vi "Shrink blobs by N pixels.vi"(8 "error in (no error)":errorcluster, 9 "Pixels to shrink":dbl=10.0, 11 "Image In":T1) -> (0 "error out":errorcluster, 3 "Image out":T1)   [LabVIEW 2013]
doc: "This vi uses a Daniellson tranfomation of the drop binary image followed by a threshold to shrink the diameter of the drop mask. Any point originally part of the mask that is within \"pixels to shrink\" of the boarder is removed from the drop mask out."
uses:
  <vilib>/vision/Image Controls.llb/IMAQ Image.ctl
  <vilib>/vision/NI_Vision_Development_Module.lvlib
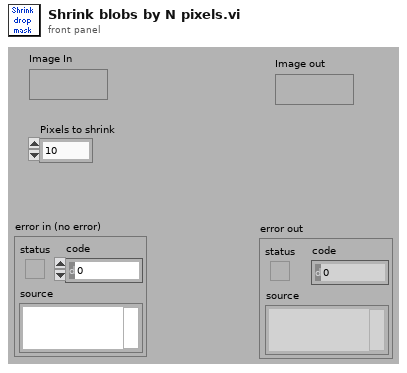
[diagram p1: front panel]
types:
  T1 = typedef "IMAQ Image.ctl" = refnum<image>
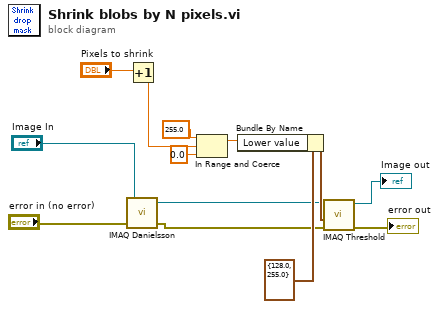
[diagram p0: block diagram]
diagram:
  n1 = call "IMAQ Danielsson"("error in (no error)"="error in (no error)", "Image Src"="Image In") -> ("error out"=w1:errorcluster, "Image Dst Out"=w2:T1)  [unwired: 2 in]
  n2 = Increment(x="Pixels to shrink") -> (x+1=w6:dbl)
  n3 = In Range and Coerce(upper limit=255.0, x=w6, lower limit=0.0) -> (coerced(x)=w3:dbl)  [unwired: 1 out]
  n4 = Bundle By Name(cluster=cluster{"Lower value":sgl, "Upper value":sgl} {"Lower value"=128.0, "Upper value"=255.0} ("Range"), "Lower value"=w3) -> (w8:cluster{"Lower value":sgl, "Upper value":sgl})
  n5 = call "IMAQ Threshold"("error in (no error)"=w1, "Range"=w8, "Image Src"=w2) -> ("error out"=→"error out":errorcluster, "Image Dst Out"=→"Image out":T1)  [unwired: 7 in]
